vi "Memory Game final version.vi"() -> ()   [LabVIEW 2019]
uses:
  <vilib>/numeric/Random Number (Range) U64.vi
  <vilib>/numeric/sub_Random U32.vi
panel:
  in  "Keys":T1
  out "Number of the correct dials":i32
  out "Display":u32(colorbox) caption="Sequence to memorise"
  # "Memory Mobile Game"
  # "Dial the colour shown in the display"
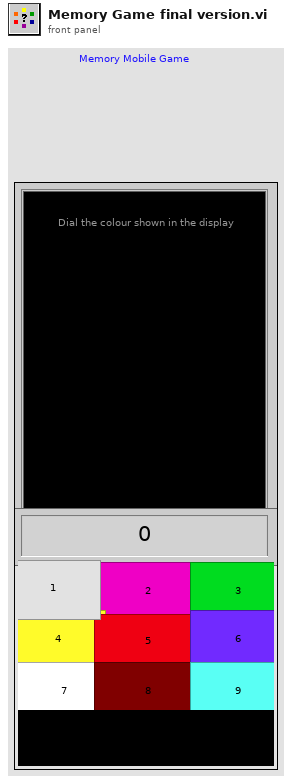
[diagram p1: front panel]
types:
  T1 = cluster{"0":bool, "1":bool, "2":bool, "3":bool, "4":bool, "5":bool, "6":bool, "7":bool, "8":bool, "9":bool}
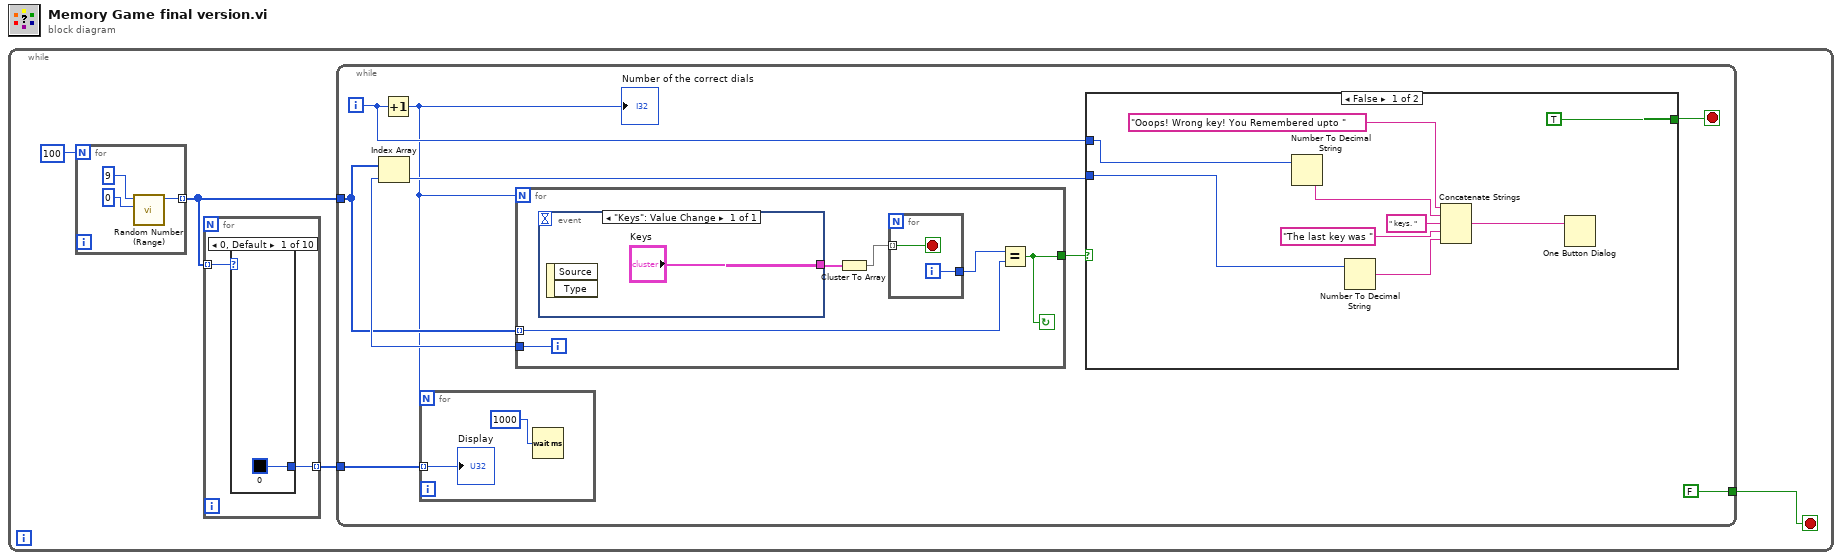
[diagram p0: block diagram]
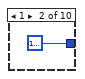
[diagram p2: hidden frame]
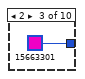
[diagram p3: hidden frame]
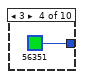
[diagram p4: hidden frame]
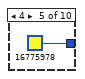
[diagram p5: hidden frame]
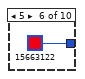
[diagram p6: hidden frame]
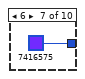
[diagram p7: hidden frame]
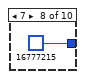
[diagram p8: hidden frame]
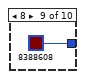
[diagram p9: hidden frame]
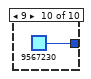
[diagram p10: hidden frame]
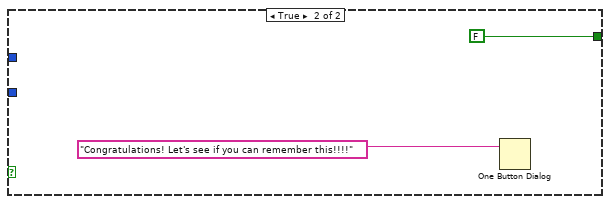
[diagram p11: hidden frame]
diagram:
  n1 = while {
    stop <- w1 stop-if-true
    # "Main loop, run  once per game"
    n2 = for {
      N: 100 -> [_]
      tunnel: [w17] -> w3 mode=indexing
      # "generate randome sequence of\ncolor indices (0 .. 9)"
      n3 = call-poly <vilib>:"Random Number (Range).vi"("lower bound (0)"=u64 0, "upper bound (100)"=u64 9) -> ("number"=w17:u64)  [unwired: 9 in]
    }
    n4 = for {
      tunnel: w3 -> [w6] mode=indexing
      tunnel: [w5] -> w2 mode=indexing
      # "generate sequence of colors"
      n5 = case shown="0, Default" w6 {
        tunnel: [u32 0 ("Color Box") u32 16777224 ("Color Box") u32 15663301 ("Color Box") u32 56351 ("Color Box") u32 16775978 ("Color Box") u32 15663122 ("Color Box") u32 7416575 ("Color Box") u32 16777215 ("Color Box") u32 8388608 ("Color Box") u32 9567230 ("Color Box")] -> w5
        frame 0, Default {
        }
        frame 1 {
        }
        frame 2 {
        }
        frame 3 {
        }
        frame 4 {
        }
        frame 5 {
        }
        frame 6 {
        }
        frame 7 {
        }
        frame 8 {
        }
        frame 9 {
        }
      }
    }
    n6 = while {
      tunnel: w3 -> [w23]
      tunnel: w2 -> [w22]
      tunnel: [FALSE] -> w1
      i -> [w25]
      stop <- w27 stop-if-true
      # "Check input of sequnece"
      n7 = Increment(x=w25) -> (x+1=w21:i32)
      "Number of the correct dials" <- w21
      n8 = for {
        N: w21 -> [_]
        tunnel: w22 -> [w29] mode=indexing
        # "play sequence"
        n9 = Wait (ms)(milliseconds to wait=u32 1000 ("Zu wartende ms")) -> ()  [unwired: 1 out]
        "Display" <- w29
      }
      n10 = for {
        N: w21 -> [_]
        tunnel: w23 -> [w44] mode=indexing
        tunnel: [w43] -> w28
        tunnel: [w42] -> w26
        i -> [w42]
        stop <- w43 continue-if-true
        # "Get and check user input"
        n11 = event shown="[0] \"Keys\": Value Change" {
          selector: _ -> [_]
          dyn-events: _ -> [_]
          timeout: _ -> [_]
          tunnel: ["Keys"] -> w47
          event "Keys": Value Change {
            n12 = event-data() -> ()  [unwired: 1 in, 2 out]
          }
        }
        n13 = Cluster To Array(cluster=w47) -> (array=w46:bool[])
        n14 = for {
          tunnel: w46 -> [w49] mode=indexing
          tunnel: [w48] -> w45
          i -> [w48]
          stop <- w49 stop-if-true
        }
        n15 = Equal?(x=w45, y=w44) -> (x = y?=w43:bool)
      }
      n16 = Index Array "Index Array"(array=w23, index=w26) -> (element=w24:u64)
      n17 = case shown="False" w28 {
        tunnel: w25 -> [w36 _]
        tunnel: [TRUE FALSE] -> w27
        tunnel: w24 -> [w33 _]
        frame False {
          # "Output message"
          n18 = Number To Decimal String(number=w36) -> (decimal integer string=w39:string)  [unwired: 1 in]
          n19 = Number To Decimal String(number=w33) -> (decimal integer string=w32:string)  [unwired: 1 in]
          n20 = Concatenate Strings "Concatenate Strings"("Ooops! Wrong key! You Remembered upto " ("message"), w39, " keys. ", "The last key was ", w32) -> (w35:string)
          n21 = One Button Dialog(message=w35) -> ()  [unwired: 1 in, 1 out]
        }
        frame True {
          n22 = One Button Dialog(message="Congratulations! Let's see if you can remember this!!!!") -> ()  [unwired: 1 in, 1 out]
        }
      }
    }
  }
